vi "Calc_sub.vi"(3 "열거형":T1(ring), 4 "B":dbl, 5 "A":dbl) -> (0 "숫자형 컨트롤":dbl, 1 "문자열":string)   [LabVIEW 2018]
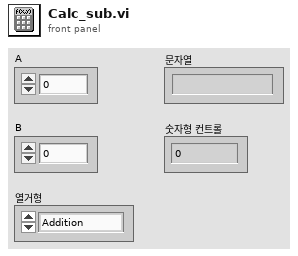
[diagram p1: front panel]
types:
  T1 = enum16{"Addition", "Subtract", "Division", "Multiply"}
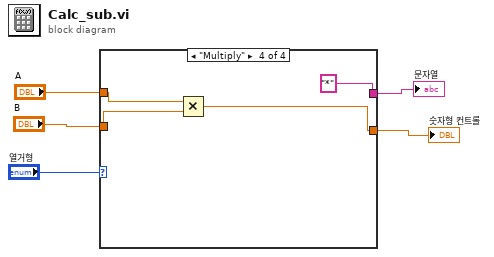
[diagram p0: block diagram]
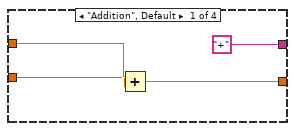
[diagram p2: hidden frame]
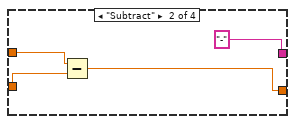
[diagram p3: hidden frame]
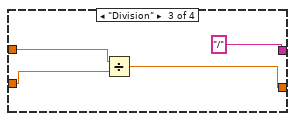
[diagram p4: hidden frame]
diagram:
  n1 = case shown="\"Multiply\"" "열거형" {
    tunnel: "A" -> [w9 w13 w17 w20]
    tunnel: "B" -> [w8 w12 w16 w19]
    tunnel: [w7 w11 w15 w18] -> w5
    tunnel: ["+" "-" "/" "*"] -> w4
    frame "Addition", Default {
      n2 = Add(x=w9, y=w8) -> (x+y=w7:dbl)
    }
    frame "Subtract" {
      n3 = Subtract(x=w13, y=w12) -> (x-y=w11:dbl)
    }
    frame "Division" {
      n4 = Divide(x=w17, y=w16) -> (x/y=w15:dbl)
    }
    frame "Multiply" {
      n5 = Multiply(x=w20, y=w19) -> (x*y=w18:dbl)
    }
  }
  "숫자형 컨트롤" <- w5
  "문자열" <- w4
